vi "LOG Loop.vi"(7 "Log Exit":refnum<notifier>, 8 "error in (no error)":errorcluster, 10 "PLC Queue in":refnum<queue>, 11 "Log Queue in":refnum<queue>) -> (0 "error out":errorcluster)   [LabVIEW 2015, in "Logger.lvlib"]
uses:
  Logger.lvlib
  support/Message Queue/Message Queue.lvlib
  TypeDefs/Logger State.ctl
  TypeDefs/Logger Data.ctl
  PL Model/API/Get Model Status Control.ctl
  PL Model/PL Model.lvlib
  <vilib>/ErrorRing/Error Ring.xnode
  support/Message Queue/Enqueue Message (Single).vi
  <vilib>/Utility/error.llb/Error Cluster From Error Code.vi
  Report/Report.lvlib
  Report/TypeDefs/Report state.ctl
  support/Message Queue/Message Cluster.ctl
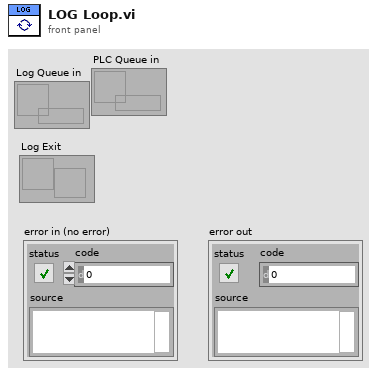
[diagram p1: front panel]
types:
  T1 = typedef "Logger.lvlib/Logger Data.ctl" = cluster{"tdms file out":refnum<k34>, "State":T2, "Path":path}
  T2 = typedef "Logger.lvlib/Logger State.ctl" = enum16{"Idle", "Working"}
  T3 = enum16{"open", "open or create", "create or replace", "create", "open (read-only)"}
  T4 = typedef "Report.lvlib/Report state.ctl" = enum16{"Create report", "Save data", "Save report", "Available printers", "Print report", "Close report"}
  T5 = typedef "PL Model.lvlib/Get Model Status Control.ctl" = cluster{"Position":dbl, "Pump State":bool, "Fluid Flow":dbl, "Fluid Level":dbl, "Barrel Number":i32, "Spill Alarm":bool, "Level Alarm":bool}
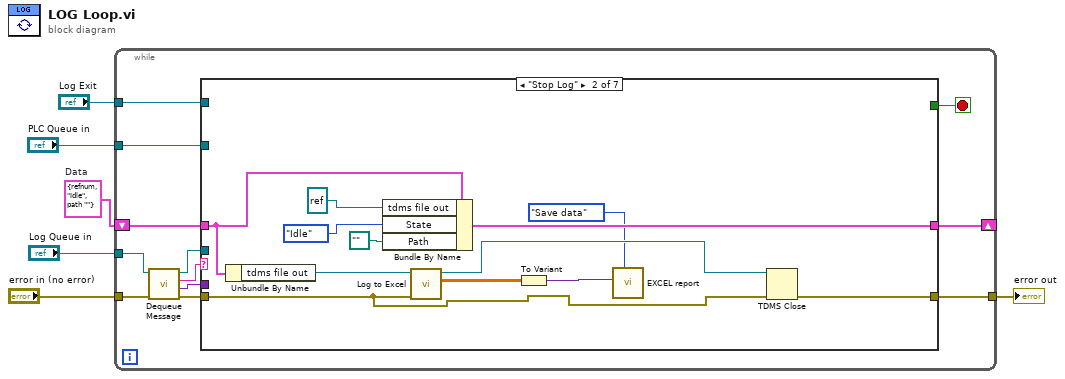
[diagram p0: block diagram]
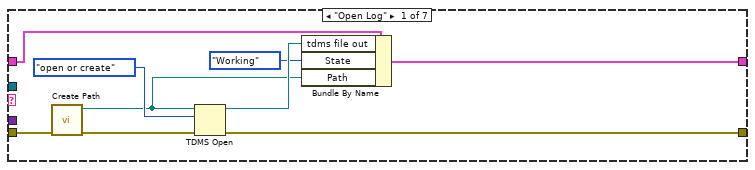
[diagram p2: hidden frame]
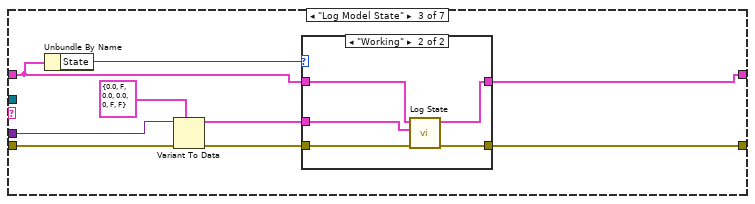
[diagram p3: hidden frame]
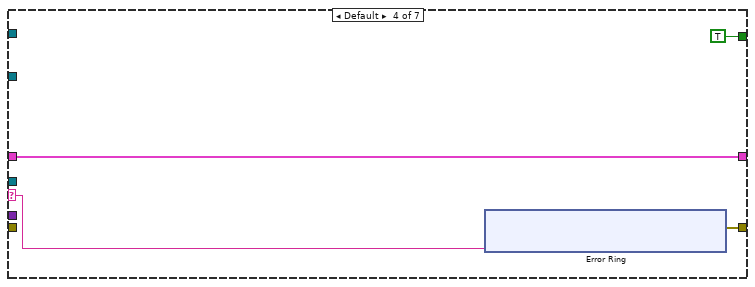
[diagram p5: hidden frame]
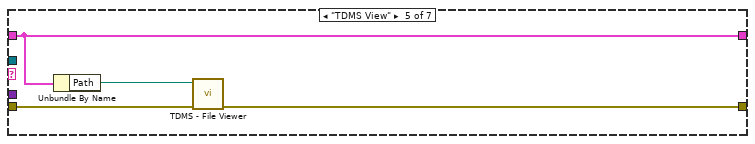
[diagram p6: hidden frame]
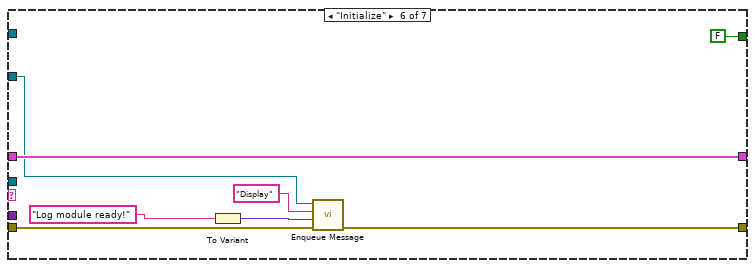
[diagram p7: hidden frame]
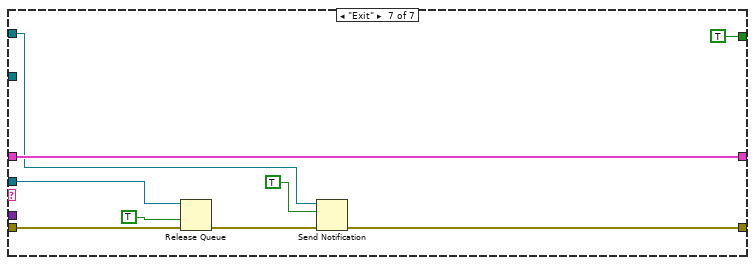
[diagram p8: hidden frame]
diagram:
  w5 = T1 {"tdms file out"=refnum, "State"=enum."Idle", "Path"=path ""}  # Data
  n1 = while {
    tunnel: "error in (no error)" -> [w18]
    tunnel: "Log Queue in" -> [w17]
    tunnel: [w12] -> w4
    shift-right: [w9] -> _
    shift-left: w5 -> [w10]
    tunnel: "Log Exit" -> [w8]
    tunnel: "PLC Queue in" -> [w7]
    stop <- w11 stop-if-true
    n2 = call "Dequeue Message.vi"("error in (no error)"=w18, "Message Queue"=w17) -> ("error out"=w16:errorcluster, "Message Data"=w13:variant, "Message"=w15:string, "dup Message Queue"=w14:refnum<queue>)  [unwired: 6 in]
    n3 = case shown="\"Stop Log\"" w15 {
      selector: w15 -> [_ _ _ w57 _ _ _]
      tunnel: w16 -> [w23 w28 w48 _ w69 w73 w84]
      tunnel: w14 -> [_ _ _ _ _ _ w83]
      tunnel: w13 -> [_ _ w46 _ _ _ _]
      tunnel: [w27 w39 w43 w56 w68 w72 w85] -> w12
      tunnel: [_ _ _ TRUE _ FALSE TRUE] -> w11
      tunnel: w10 -> [w26 w38 w41 w59 w67 w77 w87]
      tunnel: [w24 w37 w42 w59 w67 w77 w87] -> w9
      tunnel: w8 -> [_ _ _ _ _ _ w79]
      tunnel: w7 -> [_ _ _ _ _ w71 _]
      frame "Open Log" {
        n4 = call "Create Path.vi"("error in (no error)"=w23) -> ("error out"=w22:errorcluster, "File Path Control"=w19:path)  [unwired: 9 in]
        n5 = TDMS Open(8:w22, 10:T3."open or create" ("operation (0:open)"), 11:w19) -> (0:w27:errorcluster, 3:w25:refnum<k34>)  [unwired: 4 in]
        n6 = Bundle By Name(cluster=w26, "tdms file out"=w25, "State"=Logger_State."Working", "Path"=w19) -> (w24:T1)
      }
      frame "Stop Log" {
        n7 = Unbundle By Name(w38) -> ("tdms file out"=w34:refnum<k34>)
        n8 = Bundle By Name(cluster=w38, "tdms file out"=refnum<k34> refnum, "State"=Logger_State."Idle", "Path"=path "") -> (w37:T1)
        n9 = call "Log to Excel.vi"("error in"=w28, "tdms file in"=w34) -> ("appended array"=w30:dbl[][][], "tdms file out"=w33:refnum<k34>)  [unwired: 7 in, 1 out]
        n10 = To Variant(anything=w30) -> (Variant=w29:variant)
        n11 = call "EXCEL report.vi"("Report state"=Report_state."Save data", "Data in"=w29) -> ()  [unwired: 8 in, 2 out]
        n12 = TDMS Close(8:w28, 11:w33) -> (0:w39:errorcluster)  [unwired: 1 out]
      }
      frame "Log Model State" {
        n13 = Unbundle By Name(w41) -> ("State"=w40:T2)
        n14 = Variant To Data(error in=w48, type=T5 {"Position"=0.0, "Pump State"=FALSE, "Fluid Flow"=0.0, "Fluid Level"=0.0, "Barrel Number"=0, "Spill Alarm"=FALSE, "Level Alarm"=FALSE} ("Model Status"), Variant=w46) -> (data=w45:T5, error out=w44:errorcluster)
        n15 = case shown="\"Working\"" w40 {
          tunnel: w45 -> [_ w55]
          tunnel: w44 -> [w49 w54]
          tunnel: [w49 w51] -> w43
          tunnel: [w50 w52] -> w42
          tunnel: w41 -> [w50 w53]
          frame Default {
          }
          frame "Working" {
            n16 = call "Log State.vi"("error in (no error)"=w54, "Model Status"=w55, "Data"=w53) -> ("error out"=w51:errorcluster, "Data out"=w52:T1)  [unwired: 7 in]
          }
        }
      }
      frame Default {
        n17 = xnode "Error Ring"("parameter 0"=w57) -> ("error out"=w56:errorcluster)
      }
      frame "TDMS View" {
        n18 = Unbundle By Name(w67) -> ("Path"=w70:path)
        n19 = call <vilib>:"TDMS - File Viewer.vi"("error in (no error)"=w69, "file path"=w70) -> ("error out"=w68:errorcluster)  [unwired: 4 in, 1 out]
      }
      frame "Initialize" {
        n20 = To Variant(anything="Log module ready!" ("Message")) -> (Variant=w74:variant)
        n21 = call-poly "Enqueue Message.vi"("error in (no error)"=w73, "Message Data"=w74, "Message"="Display", "Message Queue"=w71) -> ("error out"=w72:errorcluster)  [unwired: 6 in, 1 out]
      }
      frame "Exit" {
        n22 = Release Queue(queue=w83, force destroy? (F)=TRUE, error in (no error)=w84) -> (error out=w82:errorcluster)  [unwired: 2 out]
        n23 = Send Notification(notification=TRUE, notifier=w79, error in (no error)=w82) -> (error out=w85:errorcluster)  [unwired: 1 out]
      }
    }
  }
  "error out" <- w4
